vi "Write Backlight.vi"(8 "error in (no error)":errorcluster, 9 "Backlight On":bool, 10 "Session In":refnum<class "Session.lvclass">, 11 "PCF8574 I2C LCD I in":refnum<class "PCF8574 I2C LCD.lvclass">) -> (0 "error out":errorcluster, 2 "Session Out":refnum<class "Session.lvclass">, 3 "PCF8574 I2C LCD I out":refnum<class "PCF8574 I2C LCD.lvclass">)   [LabVIEW 2020, in "CTI-Peripheral.lvlib" / "PCF8574 I2C LCD.lvclass"]
uses:
  PCF8574 I2C LCD.lvclass
  CTI/Session/Session.lvclass
  PCF8574 I2C LCD.lvclass/PCF8574 I2C LCD.ctl
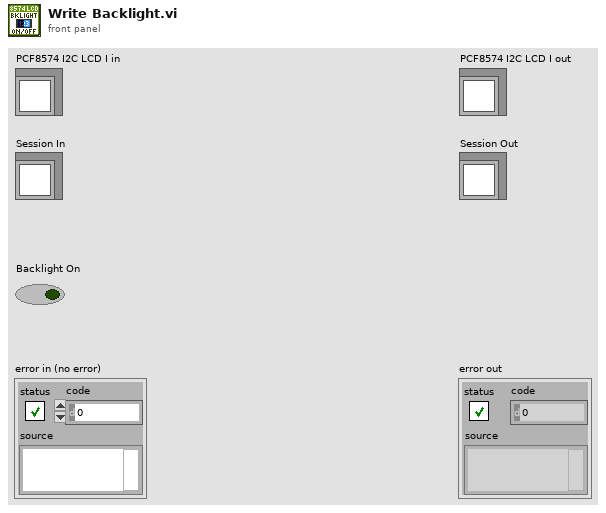
[diagram p1: front panel]
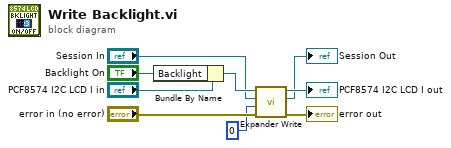
[diagram p0: block diagram]
diagram:
  n1 = Bundle By Name(cluster="PCF8574 I2C LCD I in", "Backlight"="Backlight On") -> (w5:refnum<class "PCF8574 I2C LCD.lvclass">)
  n2 = call "Expander Write.vi"("error in (no error)"="error in (no error)", "Value"=u8 0, "Session in"="Session In", "PCF8574 I2C LCD in"=w5) -> ("error out"=→"error out":errorcluster, "Session out"=→"Session Out":refnum<class "Session.lvclass">, "PCF8574 I2C LCD out"=→"PCF8574 I2C LCD I out":refnum<class "PCF8574 I2C LCD.lvclass">)  [unwired: 5 in]
